vi "Read InstrumentData.vi"(8 "error in (no error)":errorcluster, 11 "InstrumentData in":refnum<class "InstrumentData.lvclass">) -> (0 "error out":errorcluster, 2 "InstrumentData":T1, 3 "InstrumentData out":refnum<class "InstrumentData.lvclass">)   [LabVIEW 2023, in "InstrumentData.lvclass"]
uses:
  InstrumentData.lvclass
  typedefs/InstrumentData.ctl
  typedefs/instrumentType.ctl
  InstrumentData.lvclass/InstrumentData.ctl
  typedefs/typedefs.lvlib
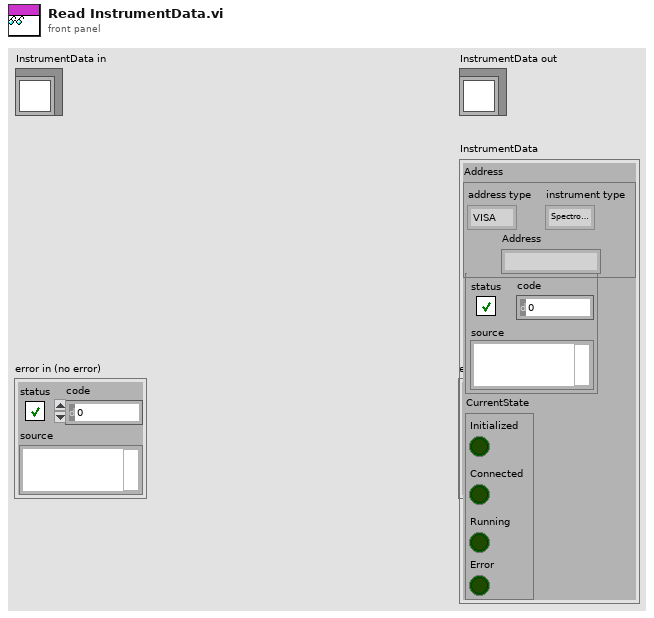
[diagram p1: front panel]
types:
  T1 = typedef "typedefs.lvlib/InstrumentData.ctl" = cluster{"Instr Error":errorcluster, "Address":cluster{"address type":enum16{"VISA", "Index"}, "Address":string, "instrument type":T2}, "CurrentState":cluster{"Initialized":bool, "Connected":bool, "Running":bool, "Error":bool}}
  T2 = typedef "typedefs.lvlib/instrumentType.ctl" = enum16{"Spectrometer", "Camera", "Stepper", "Piezo"}
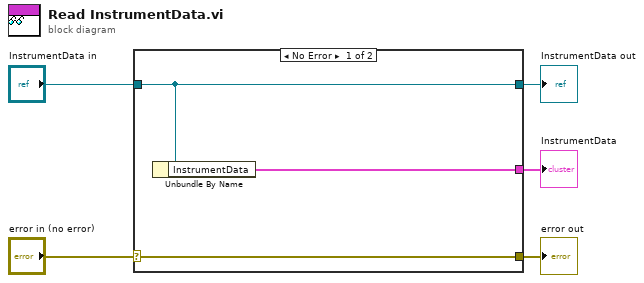
[diagram p0: block diagram]
diagram:
  n1 = case shown="No Error" "error in (no error)" {
    selector: "error in (no error)" -> [w8 w9]
    tunnel: [w8 w9] -> w4
    tunnel: [w7 w10] -> w2
    tunnel: "InstrumentData in" -> [w7 w10]
    tunnel: [w6 _] -> w1
    frame No Error {
      n2 = Unbundle By Name(w7) -> ("InstrumentData"=w6:T1)
    }
    frame Error {
    }
  }
  "error out" <- w4
  "InstrumentData out" <- w2
  "InstrumentData" <- w1
